vi "FreeGPUImage.vi"(0 "GPU Image Pointer":u64) -> ()   [LabVIEW 2011]
uses:
  cudatrack-debug.dll
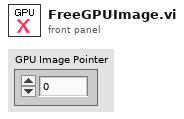
[diagram p1: front panel]
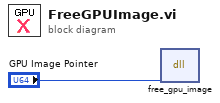
[diagram p0: block diagram]
diagram:
  n1 = dll-call lib="D:/jcnossen1/cudaqi-tracker/cudaqi/cudatrack-debug.dll" fn="free_gpu_image"("image"="GPU Image Pointer") -> ()  [unwired: 5 in, 2 out]
